vi "INIT.vi"(8 "error in (no error)":errorcluster, 11 "Actor_USD in":refnum<class "Actor_USD.lvclass">) -> (0 "error out":errorcluster, 3 "Actor_USD out":refnum<class "Actor_USD.lvclass">)   [LabVIEW 2019, in "Actor_USD.lvlib" / "Actor_USD.lvclass"]
uses:
  Actor_USD.lvclass
  Actor_USD.lvclass/Actor_USD.ctl
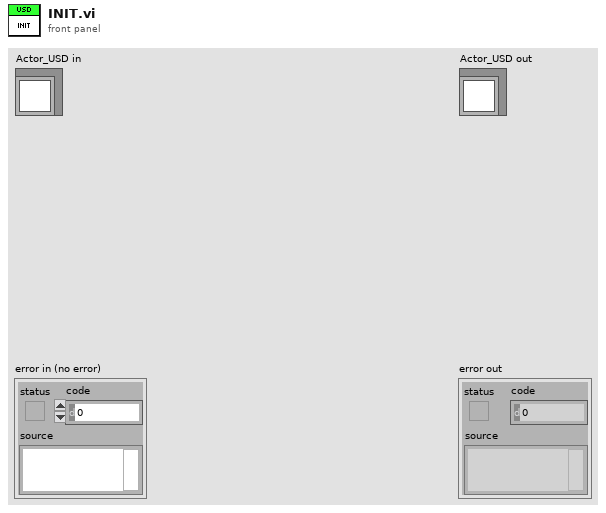
[diagram p1: front panel]
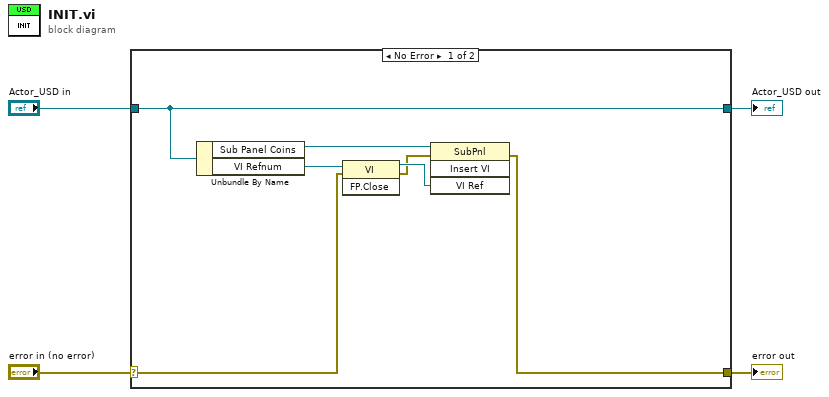
[diagram p0: block diagram]
diagram:
  n1 = case shown="No Error" "error in (no error)" {
    selector: "error in (no error)" -> [w6 w13]
    tunnel: [w5 w13] -> w3
    tunnel: [w7 w12] -> w1
    tunnel: "Actor_USD in" -> [w7 w12]
    frame No Error {
      n2 = Unbundle By Name(w7) -> ("Sub Panel Coins"=w10:refnum<vi>, "VI Refnum"=w11:refnum<vi>)
      n3 = invoke class="VI" method="FP.Close"(reference=w11, error in=w6) -> (reference out=w9:refnum<vi>, error out=w8:errorcluster)  [unwired: 1 in, 1 out]
      n4 = invoke class="SubPnl" method="Insert VI"(reference=w10, error in=w8, "VI Ref"=w9) -> (error out=w5:errorcluster)  [unwired: 1 in, 3 out]
    }
    frame Error {
    }
  }
  "error out" <- w3
  "Actor_USD out" <- w1
